vi "CheckLimit.vi"(3 "note":string, 8 "high":dbl, 9 "low":dbl, 10 "value":dbl, 11 "step name":string) -> (5 "margin":dbl, 6 "Result":T1, 7 "pass led":bool)   [LabVIEW 2026]
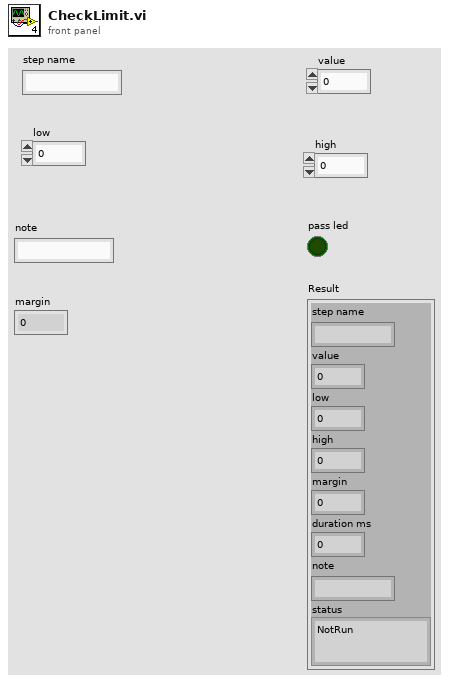
[diagram p1: front panel]
types:
  T1 = cluster{"step name":string, "value":dbl, "low":dbl, "high ":dbl, "margin":dbl, "duration ms":dbl, "note":string, "status":enum16{"NotRun", "Pass", "Fail", "Skipped"}}
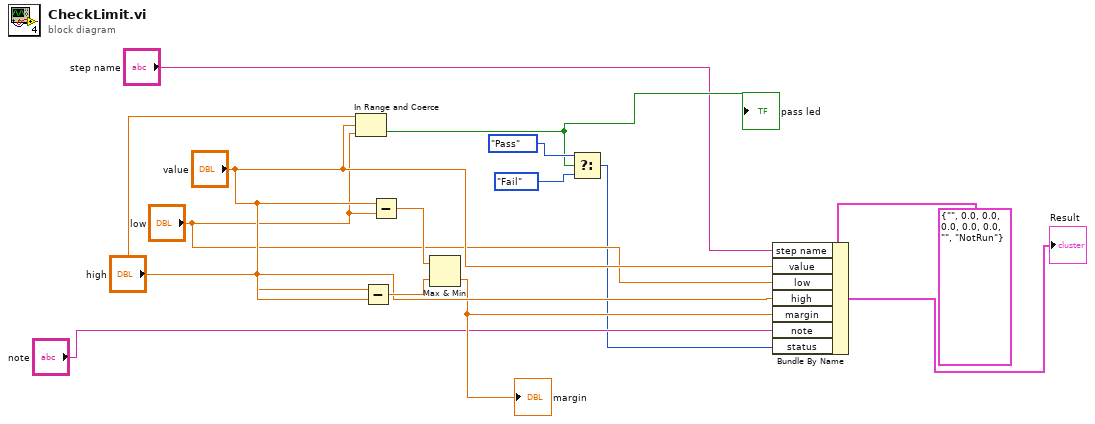
[diagram p0: block diagram]
diagram:
  n1 = In Range and Coerce(upper limit="high", x="value", lower limit="low") -> (In Range?=w10:bool)  [unwired: 1 out]
  "pass led" <- w10
  n2 = Subtract(x="high", y="value") -> (x-y=w13:dbl)
  n3 = Subtract(x="value", y="low") -> (x-y=w14:dbl)
  n4 = Max & Min(x=w14, y=w13) -> (min(x,y)=w4:dbl)  [unwired: 1 out]
  "margin" <- w4
  n5 = Select(t=enum16{"NotRun", "Pass", "Fail", "Skipped"}."Pass" ("Enum"), s=w10, f=enum16{"NotRun", "Pass", "Fail", "Skipped"}."Fail" ("Enum")) -> (s? t:f=w2:enum16{"NotRun", "Pass", "Fail", "Skipped"})
  n6 = Bundle By Name(cluster=T1 {"step name"="", "value"=0.0, "low"=0.0, "high "=0.0, "margin"=0.0, "duration ms"=0.0, "note"="", "status"=enum."NotRun"} ("Result 2"), "step name"="step name", "value"="value", "low"="low", "high"="high", "margin"=w4, "note"="note", "status"=w2) -> (→"Result":T1)
